vi "Add2Lib.vi"(4 "ProjectPath":path=path "F:/LVSCC/LV2009/GPL/lib.lib/LVOOP/HGF_MobileAgentSystem/MoAgSy_Scripting/TestAgent/TestAgent.lvproj", 6 "LibraryPath":path, 8 "error in (no error)":errorcluster, 10 "Created Classes":path[](array[path])) -> (0 "error out":errorcluster)   [LabVIEW 2009, in "HGF_VisitorGenerator.lvlib"]
doc: "add created classes to agent library"
uses:
  HGF_VisitorGenerator.lvlib
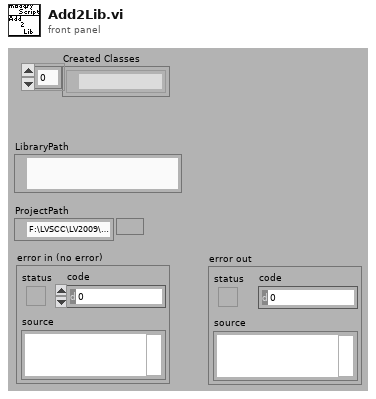
[diagram p1: front panel]
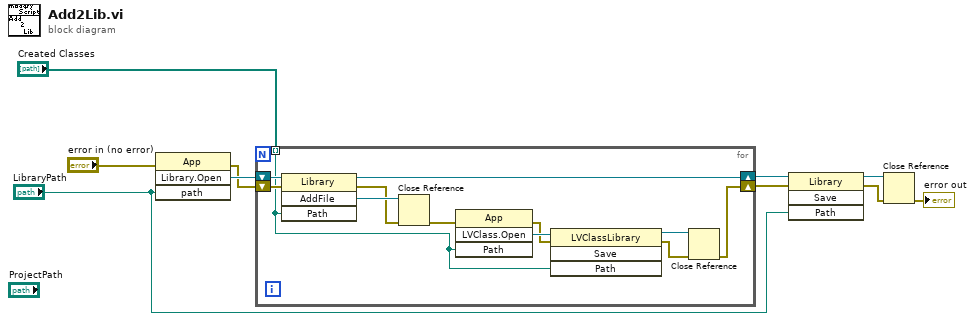
[diagram p0: block diagram]
diagram:
  n1 = invoke class="App" method="Library.Open"(error in="error in (no error)", "path"="LibraryPath") -> (error out=w8:errorcluster, "Open Library"=w10:refnum<vi>)  [unwired: 2 in, 2 out]
  n2 = for {
    tunnel: "Created Classes" -> [w16] mode=indexing
    shift-right: [w21] -> w7
    shift-left: w10 -> [w22]
    shift-right: [w11] -> w6
    shift-left: w8 -> [w20]
    n3 = invoke class="Library" method="AddFile"(reference=w22, error in=w20, "Path"=w16) -> (reference out=w21:refnum<vi>, error out=w18:errorcluster, "AddFile"=w19:refnum<vi>)  [unwired: 1 in, 1 out]
    n4 = Close Reference(reference=w19, error in (no error)=w18) -> (error out=w12:errorcluster)
    n5 = invoke class="App" method="LVClass.Open"(error in=w12, "Path"=w16) -> (error out=w15:errorcluster, "LVClass.Open"=w17:refnum<vi>)  [unwired: 2 in, 2 out]
    n6 = invoke class="LVClassLibrary" method="Save"(reference=w17, error in=w15, "Path"=w16) -> (reference out=w14:refnum<vi>, error out=w13:errorcluster)  [unwired: 1 in, 2 out]
    n7 = Close Reference(reference=w14, error in (no error)=w13) -> (error out=w11:errorcluster)
  }
  n8 = invoke class="Library" method="Save"(reference=w7, error in=w6, "Path"="LibraryPath") -> (reference out=w4:refnum<vi>, error out=w1:errorcluster)  [unwired: 1 in, 2 out]
  n9 = Close Reference(reference=w4, error in (no error)=w1) -> (error out=→"error out":errorcluster)
